vi "Get Service File Path.vi"() -> (2 "service setting file":path)   [LabVIEW 2021, in "AudioGenUtility.lvlib"]
uses:
  AudioGenUtility.lvlib
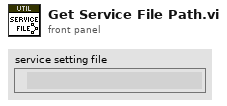
[diagram p1: front panel]
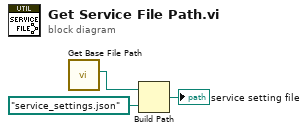
[diagram p0: block diagram]
diagram:
  n1 = call "Get Base File Path.vi"() -> ("base path"=w3:path)  [unwired: 11 in]
  n2 = Build Path(base path=w3, name or relative path=path "service_settings.json") -> (appended path=→"service setting file":path)
